vi "UserVars-Expression to Vector (V2).vi"(7 "Expr":string, 11 "error in (no error)":errorcluster) -> (8 "Values":dbl[](array[numeric]), 15 "error out":errorcluster)   [LabVIEW 2020]
uses:
  <vilib>/gmath/NI_Gmath.lvlib
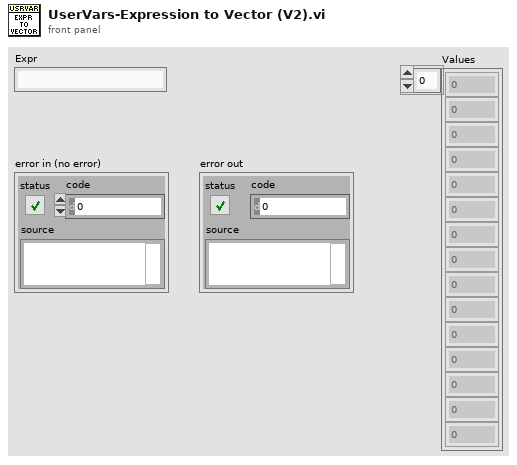
[diagram p1: front panel]
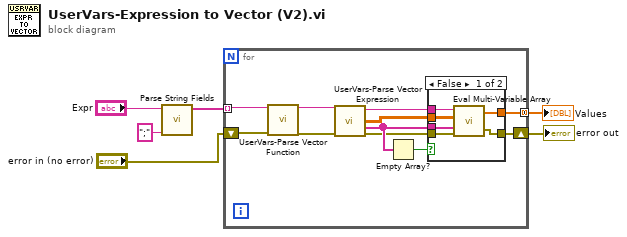
[diagram p0: block diagram]
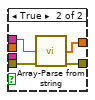
[diagram p2: hidden frame]
diagram:
  n1 = call "Parse String Fields.vi"("Separator"=";", "String"="Expr") -> ("Fields"=w1:string[])  [unwired: 8 in, 1 out]
  n2 = for {
    tunnel: [w15] -> w6 mode=concatenating
    tunnel: w1 -> [w10] mode=indexing
    shift-right: [w14] -> w5
    shift-left: "error in (no error)" -> [w7]
    n3 = call "UserVars-Parse Vector Function.vi"("Expr in"=w10, "error in (no error)"=w7) -> ("Expr out"=w9:string, "error out"=w8:errorcluster)  [unwired: 12 in]
    n4 = call "UserVars-Parse Vector Expression.vi"("Expression In"=w9, "error in (no error)"=w8) -> ("Expression Out"=w11:string, "values"=w12:dbl[][], "variables"=w16:string[], "error out"=w13:errorcluster)  [unwired: 10 in]
    n5 = Empty Array?(array=w16) -> (empty?=w17:bool)
    n6 = case shown="False" w17 {
      tunnel: w11 -> [w23 w26]
      tunnel: w12 -> [w22 _]
      tunnel: w16 -> [w21 _]
      tunnel: w13 -> [w20 w24]
      tunnel: [w19 w27] -> w14
      tunnel: [w18 w25] -> w15
      frame False {
        n7 = call <vilib>:"Eval Multi-Variable Array.vi"("error in (no error)"=w20, "Variables"=w21, "X Values"=w22, "formula"=w23) -> ("error out"=w19:errorcluster, "Y Values"=w18:dbl[])
      }
      frame True {
        n8 = call "Array-Parse from string.vi"("String"=w26, "error in (no error)"=w24) -> ("Array"=w25:dbl[], "error out"=w27:errorcluster)  [unwired: 12 in]
      }
    }
  }
  "error out" <- w5
  "Values" <- w6
